vi "FormatPercentage.vi"(10 "Precision":i16, 11 "Raw Percentage":dbl) -> (3 "Formatted Percentage":string)   [LabVIEW 2024]
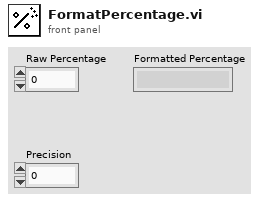
[diagram p1: front panel]
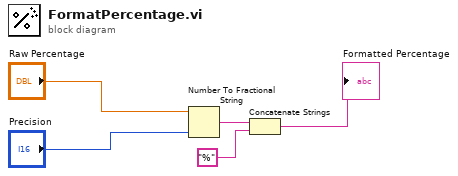
[diagram p0: block diagram]
diagram:
  n1 = Number To Fractional String(number="Raw Percentage", precision (6)="Precision") -> (F-format string=w4:string)  [unwired: 2 in]
  n2 = Concatenate Strings(w4, "%" ("string")) -> (→"Formatted Percentage":string)
